vi "serial.vi"() -> ()   [LabVIEW 2024]
uses:
  <vilib>/Instr/_visa.llb/VISA Configure Serial Port (Instr).vi
panel:
  in  "Modified Date":timestamp format="%<%d/%m/%Y>T"
  in  "Curent Date":timestamp=timestamp(3786912000 s since 1904-01-01) caption="Time Stamp" format="%<%d/%m/%Y>T"
  in  "Serial Number":u32 format="%04d"
  in  "Batch number":string
  in  "Part No":u16(ring) caption="Part Number" items=["WM08964-0002", "WM05989-0001", "WM07895-0005"]
  in  "stop":bool
  in  "Send":bool
  in  "COM Port":refnum<visa-resource-name>
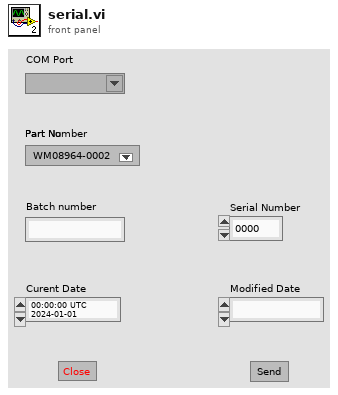
[diagram p1: front panel]
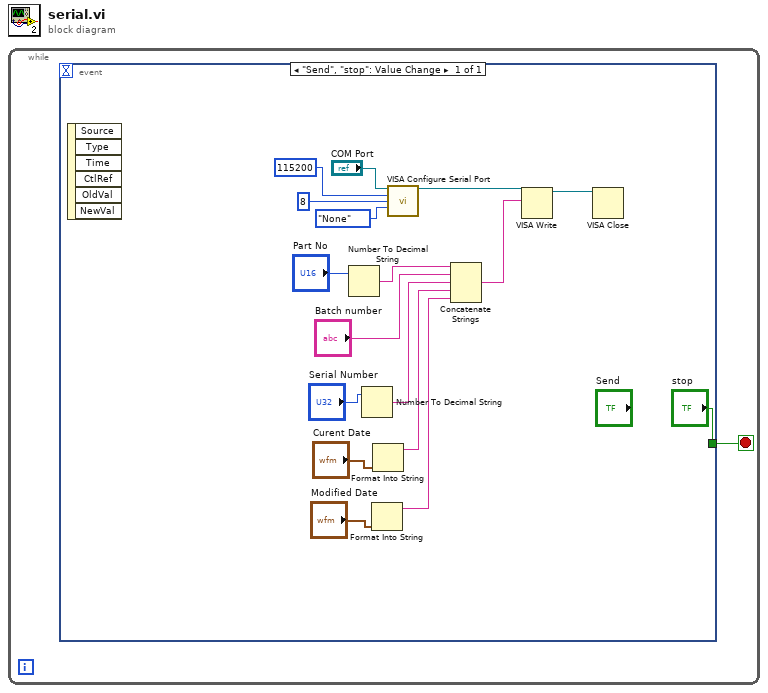
[diagram p0: block diagram]
diagram:
  n1 = while {
    stop <- w1 stop-if-true
    n2 = event shown="[0] \"Send\", \"stop\": Value Change" {
      selector: _ -> [_]
      dyn-events: _ -> [_]
      timeout: _ -> [_]
      tunnel: ["stop"] -> w1
      event "Send", "stop": Value Change {
        n3 = event-data() -> ()  [unwired: 1 in, 6 out]
        n4 = Number To Decimal String(number="Part No") -> (decimal integer string=w11:string)  [unwired: 1 in]
        n5 = Number To Decimal String(number="Serial Number") -> (decimal integer string=w6:string)  [unwired: 1 in]
        n6 = Format Into String("Modified Date") -> (resulting string=w2:string)  [unwired: 3 in, 1 out]
        n7 = Format Into String("Curent Date") -> (resulting string=w3:string)  [unwired: 3 in, 1 out]
        n8 = call-poly "VISA Configure Serial Port"("VISA resource name"="COM Port", "baud rate (9600)"=u32 115200, "data bits (8)"=u16 8, "parity (0:none)"=enum16{"None", "Odd", "Even", "Mark", "Space"}."None") -> ("VISA resource name out"=w8:refnum<visa-resource-name>)  [unwired: 10 in, 1 out]
        n9 = Concatenate Strings(w11, "Batch number", w6, w3, w2) -> (w9:string)
        n10 = VISA Write(VISA resource name=w8, write buffer=w9) -> (VISA resource name out=w13:refnum<visa-resource-name>)  [unwired: 1 in, 2 out]
        n11 = VISA Close(VISA resource name=w13) -> ()  [unwired: 1 in, 1 out]
      }
    }
  }
